vi "Accumet copyright.vi"   [LabVIEW 2010]
panel:
  # "Compumet\nData Acquisition and Control\nfor Accumet 50 meters"
  # "©2002 Monroe Weber-Shirk\nall rights reserved\nmw24@cornell.edu\nDocumentation available at:\nwww.cee.cornell.edu/mw24/software\nCivil and Environmental Engineering\nCornell University"
  # "This software may be modified as needed by the end user \nprovided this copyright dialog is included."
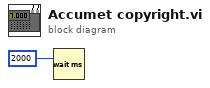
[diagram p0: block diagram]
diagram:
  n1 = Wait (ms)(milliseconds to wait=2000) -> ()  [unwired: 1 out]
